vi "Pause.vi"(8 "error in (no error)":errorcluster, 11 "Huber Settings":T1) -> (0 "error out":errorcluster, 3 "Huber Settings":T1)   [LabVIEW 2018, in "Huber Ministat 230 TCU.lvlib"]
uses:
  Huber Ministat 230 TCU.lvlib
  Huber Settings.ctl
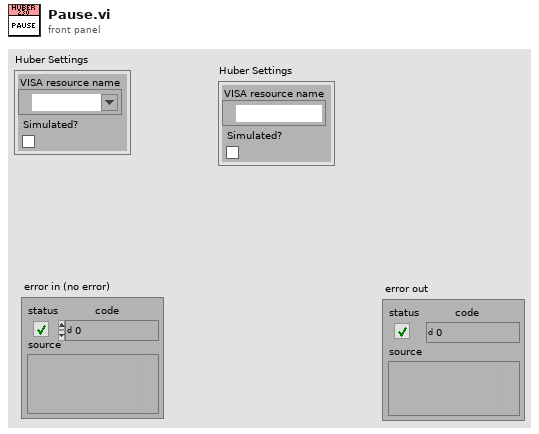
[diagram p1: front panel]
types:
  T1 = typedef "Huber Ministat 230 TCU.lvlib/Huber Settings.ctl" = cluster{"VISA resource name":refnum<visa-resource-name>, "Simulated?":bool}
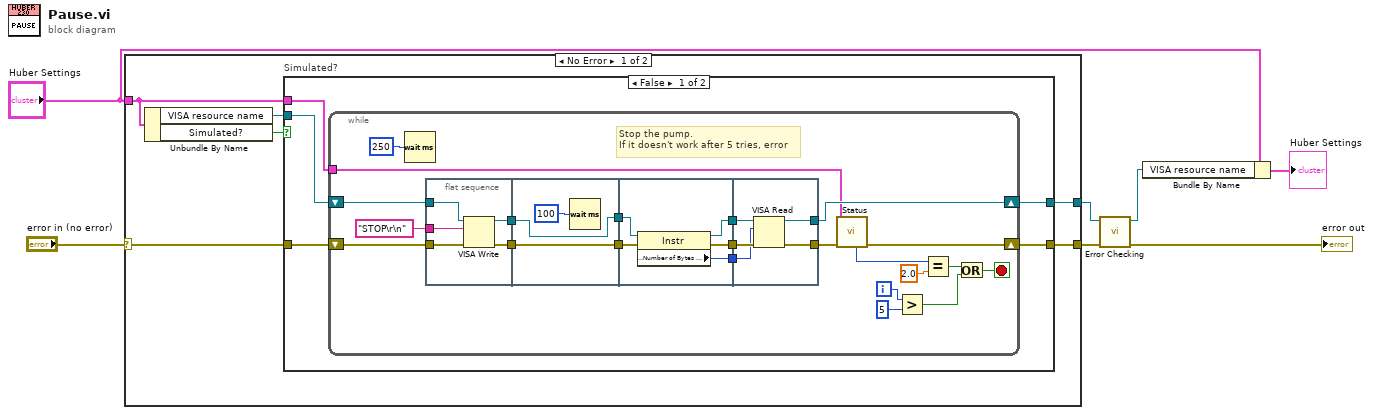
[diagram p0: block diagram]
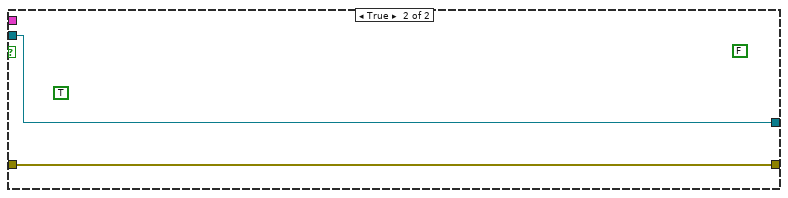
[diagram p2: hidden frame]
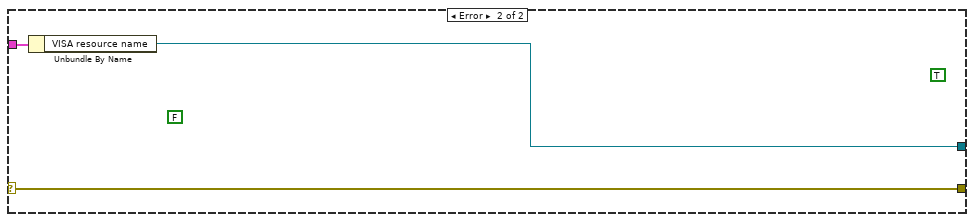
[diagram p3: hidden frame]
diagram:
  n1 = case shown="No Error" "error in (no error)" {
    selector: "error in (no error)" -> [w13 w63]
    tunnel: "Huber Settings" -> [w8 w62]
    tunnel: [w12 w63] -> w5
    tunnel: [w10 w61] -> w6
    frame No Error {
      n2 = Unbundle By Name(w8) -> ("VISA resource name"=w11:refnum<visa-resource-name>, "Simulated?"=w9:bool)
      n3 = case "Simulated?" shown="False" w9 {
        tunnel: w13 -> [w16 w60]
        tunnel: [w14 w60] -> w12
        tunnel: [w18 w59] -> w10
        tunnel: w11 -> [w17 w59]
        tunnel: w8 -> [w15 _]
        frame False {
          n4 = while {
            tunnel: w15 -> [w29]
            shift-right: [w32] -> w18
            shift-left: w17 -> [w31]
            shift-right: [w27] -> w14
            shift-left: w16 -> [w30]
            i -> [w22]
            stop <- w23 stop-if-true
            # "Stop the pump. \nIf it doesn't work after 5 tries, error"
            n5 = Wait (ms)(milliseconds to wait=u32 250) -> ()  [unwired: 1 out]
            n6 = flat-sequence {
              tunnel: "STOP\r\n" ("string") -> [w45]
              tunnel: [w44] -> w40
              tunnel: [w43] -> w39
              tunnel: w31 -> [w42]
              tunnel: w30 -> [w41]
              tunnel: w40 -> [w47]
              tunnel: w39 -> [w46]
              tunnel: [w47] -> w38
              tunnel: [w46] -> w37
              tunnel: [w51] -> w36
              tunnel: [w50] -> w35
              tunnel: [w49] -> w34
              tunnel: w38 -> [w53]
              tunnel: w37 -> [w52]
              tunnel: [w58] -> w28
              tunnel: [w57] -> w32
              tunnel: w36 -> [w56]
              tunnel: w35 -> [w55]
              tunnel: w34 -> [w54]
              frame #0 {
                n7 = VISA Write(VISA resource name=w42, write buffer=w45, error in (no error)=w41) -> (VISA resource name out=w44:refnum<visa-resource-name>, error out=w43:errorcluster)  [unwired: 1 out]
              }
              frame #1 {
                n8 = Wait (ms)(milliseconds to wait=u32 100) -> ()  [unwired: 1 out]
              }
              frame #2 {
                n9 = property class="Instr"(reference=w53, error in=w52) -> (reference out=w51:refnum<visa-resource-name>, error out=w50:errorcluster, "Serial Settings:Number of Bytes at Serial Port"=w49:u32)
              }
              frame #3 {
                n10 = VISA Read(VISA resource name=w56, byte count=w54, error in (no error)=w55) -> (VISA resource name out=w57:refnum<visa-resource-name>, error out=w58:errorcluster)  [unwired: 2 out]
              }
            }
            n11 = call "Status.vi"("error in (no error)"=w28, "Huber Settings"=w29) -> ("error out"=w27:errorcluster, "Temp"=w25:i32)  [unwired: 5 in, 3 out]
            n12 = Greater?(x=w22, y=5) -> (0:w20:bool)
            n13 = Equal?(x=w25, y=2.0) -> (x = y?=w24:bool)
            n14 = Or(x=w24, y=w20) -> (x .or. y?=w23:bool)
          }
        }
        frame True {
          (unwired) TRUE
          (unwired) FALSE
        }
      }
    }
    frame Error {
      (unwired) FALSE
      (unwired) TRUE
      n15 = Unbundle By Name(w62) -> ("VISA resource name"=w61:refnum<visa-resource-name>)
    }
  }
  n16 = call "Error Checking.vi"("error in (no error)"=w5, "VISA resource name"=w6) -> ("error out"=→"error out":errorcluster, "VISA resource name"=w3:refnum<visa-resource-name>)  [unwired: 7 in, 1 out]
  n17 = Bundle By Name(cluster="Huber Settings", "VISA resource name"=w3) -> (→"Huber Settings":T1)
